vi "string_2_enum.vi"() -> ()   [LabVIEW 2013]
uses:
  thcd_controls/ctrl_uom_thcd.ctl
panel:
  out "Strings []":string[](array[string])
  out "uom 2":T1
  out "uom":T1
  in  "input string":string
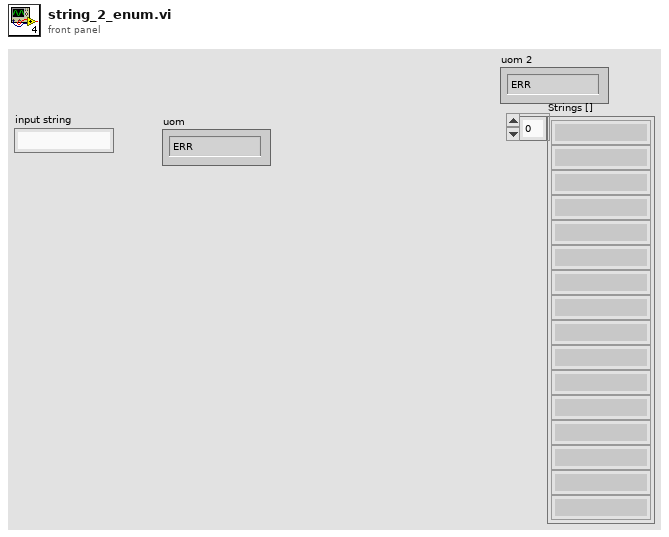
[diagram p1: front panel]
types:
  T1 = typedef "ctrl_uom_thcd.ctl" = enum16{"ERR", "SCCM", "SLM", "%", "V", "MV", "CNT", "NLM", "SLS", "NLS", "SLH", "NLH", "SMLM", "NMLM", "SMLS", "NMLS", "SMLH", "NMLH", "NCCM", "SCCS", "NCCS", "SCCH", "NCCH", "SCFM", "NCFM", "SCFS", "NCFS", "SCFH", "NCFH", "SCMM", "NCMM", "SCMS", "NCMS", "SCMH", "NCMH", "SCIM", "NCIM", "SCIS", "NCIS", "SCIH", "NCIH", "LBM", "LBS", "LBH", "KgM", "KgS", "KgH", "GRM", "GMS", "GRH", "MolM", "MolS", "MolH", "KMolM", "KMolS", "KMolH", "W", "BPS", "Sec", "Min", "Hrs", "WH", "Torr", "Bar", "Pa", "inH2O", "PSIA", "PSIG"}
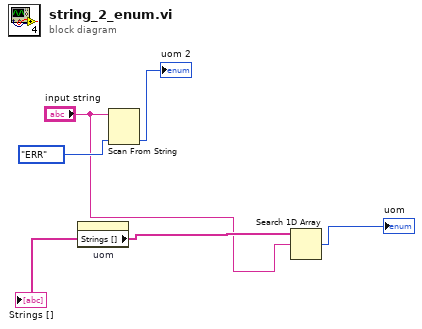
[diagram p0: block diagram]
diagram:
  n1 = property on="uom" class="Enum (strict)"() -> ("Strings []"=w4:string[])  [unwired: 2 in, 2 out]
  "Strings []" <- w4
  n2 = Scan From String(input string="input string", default 1=ctrl_uom_thcd."ERR" ("uom 2")) -> (output 1=→"uom 2":T1)  [unwired: 3 in, 3 out]
  n3 = Search 1D Array(1D array=w4, element="input string") -> (index of element=→"uom":i32)  [unwired: 1 in]
